vi "Shoot Fuel.vi"(11 "Input Velocities":T1) -> (2 "Hood Setpoint":dbl, 3 "Shooter RPM":dbl)   [LabVIEW 2025]
uses:
  swerve-template/Type Definitions/Data/Robot Velocities.ctl
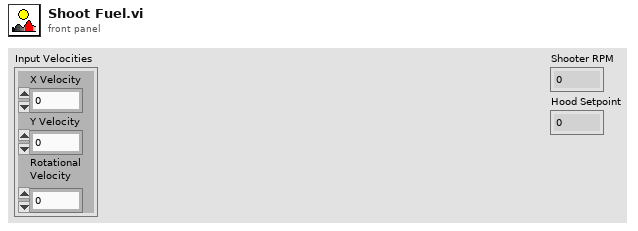
[diagram p1: front panel]
types:
  T1 = typedef "Robot Velocities.ctl" = cluster{"X Velocity":dbl, "Y Velocity":dbl, "Rotational \nVelocity":dbl}
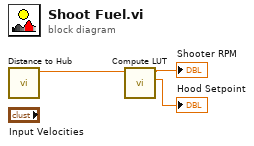
[diagram p0: block diagram]
diagram:
  n1 = call "Distance to Hub.vi"() -> ("Distance to Hub (ft)"=w2:dbl)  [unwired: 10 in, 1 out]
  n2 = call "Compute LUT.vi"("Hub Distance (ft)"=w2) -> ("Hood Setpoint"=→"Hood Setpoint":dbl, "Shooter RPM"=→"Shooter RPM":dbl)  [unwired: 9 in]
